vi "Teleop.vi"(10 "Match Info":T1={"Autonomous Elapsed Seconds"=0.0, "TeleOp Elapsed Seconds"=0.0, "Disabled Elapsed Seconds"=0.0, "Visited Autonomous"=FALSE, "Visited TeleOp"=FALSE, "Visited Disabled"=FALSE, "Autonomous Settings"={"Autonomous Style"=enum."Independent", "VI Refnum"=refnum}}, 11 "Call Context":T2) -> ()   [LabVIEW 2020]
doc: "This VI is called for each enabled TeleOp packet received from the DS. It is typically used to read from joysticks and other inputs and update I/O or setpoints for timed control loops. It should complete and return within 20 milliseconds or risk missing DS packets."
uses:
  <vilib>/Rock Robotics/WPI/DriverStation/WPI_DriverStationDerivedRobotMode.ctl
  <vilib>/Rock Robotics/WPI/DriverStation/WPI_DriverStationMatch Info.ctl
  <vilib>/Rock Robotics/WPI/ThirdParty/REV Robotics/REVLib/Typedef/Spark MAX Control Type.ctl
  <vilib>/Rock Robotics/WPI/Utilities/WPI_GetSetVariantRefNum.vi
  <vilib>/Rock Robotics/Network Tables/NT Write Boolean Array.vi
  <vilib>/Rock Robotics/Network Tables/NT Write Numeric Array.vi
  Framework/Robot Global Data.vi
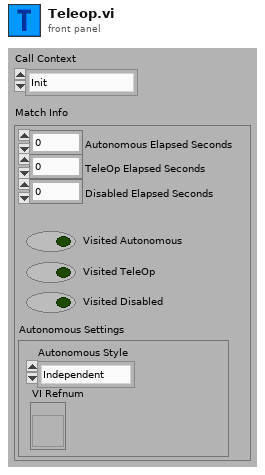
[diagram p1: front panel]
types:
  T1 = typedef "WPI_DriverStationMatch Info.ctl" = cluster{"Autonomous Elapsed Seconds":dbl, "TeleOp Elapsed Seconds":dbl, "Disabled Elapsed Seconds":dbl, "Visited Autonomous":bool, "Visited TeleOp":bool, "Visited Disabled":bool, "Autonomous Settings":cluster{"Autonomous Style":enum16{"Iterative", "Independent"}, "VI Refnum":refnum<vi>}}
  T2 = typedef "WPI_DriverStationDerivedRobotMode.ctl" = enum16{"Init", "Execute", "Stop"}
  T3 = typedef "Spark MAX Control Type.ctl" = enum16{"Percent VBus", "Voltage", "Velocity", "Position", "Smart Motion", "Current", "Smart Velocity"}
  T4 = typedef "WPI_JoystickDevRef.ctl" = cluster{"Device":T5}
  T5 = typedef "WPI_JoystickDeviceEnum.ctl" = enum16{"USB 0", "USB 1", "USB 2", "USB 3", "USB 4", "USB 5"}
  T6 = typedef "Command Status Info.ctl" = cluster{"Name":string, "Status":T7, "notifier out":T8}
  T7 = typedef "Completion Status.ctl" = enum16{"Successful", "Aborted", "Incomplete"}
  T8 = typedef "Completion Notifier.ctl" = refnum<notifier>
  T9 = typedef "WPI_MotorControlDeviceRef.ctl" = cluster{"DeviceStatus":errorcluster, "Type":T10, "PWM":cluster{"PWM Channel":T11, "DeadBand":T12}, "CAN":cluster{"Device Number":u8, "SetOutput VI Ref":variant, "GetOutput VI Ref":variant, "Enable VI Ref":variant, "Disable VI Ref":variant, "Data":variant}, "Invert":bool, "DIO PWM":cluster{"PWM \"Enable\" Channel":T11, "DIOChannel":T13, "PWM Rate":dbl}}
  T10 = typedef "WPI_MotorControlType.ctl" = enum16{"PWM", "CAN", "DIO PWM"}
  T11 = typedef "FPGA_DIOPWMChannel.ctl" = enum8{"PWM 0", "PWM 1", "PWM 2", "PWM 3", "PWM 4", "PWM 5", "PWM 6", "PWM 7", "PWM 8", "PWM 9", "PWM MXP 0", "PWM MXP 1", "PWM MXP 2", "PWM MXP 3", "PWM MXP 4", "PWM MXP 5", "PWM MXP 6", "PWM MXP 7", "PWM MXP 8", "PWM MXP 9", "Invalid"}
  T12 = typedef "WPI_PWMDeadband.ctl" = cluster{"Name":string, "maxPositivePwm":i32, "minPositivePwm":i32, "centerPwm":i32, "maxNegativePwm":i32, "minNegativePwm":i32, "angularRange":u16}
  T13 = typedef "FPGA_DIOChannel.ctl" = enum8{"DIO 0", "DIO 1", "DIO 2", "DIO 3", "DIO 4", "DIO 5", "DIO 6", "DIO 7", "DIO 8", "DIO 9", "DIO MXP 0", "DIO MXP 1", "DIO MXP 2", "DIO MXP 3", "DIO MXP 4", "DIO MXP 5", "DIO MXP 6", "DIO MXP 7", "DIO MXP 8", "DIO MXP 9", "DIO MXP 10", "DIO MXP 11", "DIO MXP 12", "DIO MXP 13", "DIO MXP 14", "DIO MXP 15", "SPI Port CS1", "SPI Port CS2", "SPI Port CS3", "SPI Port MISO", "SPI Port MOSI", "Invalid"}
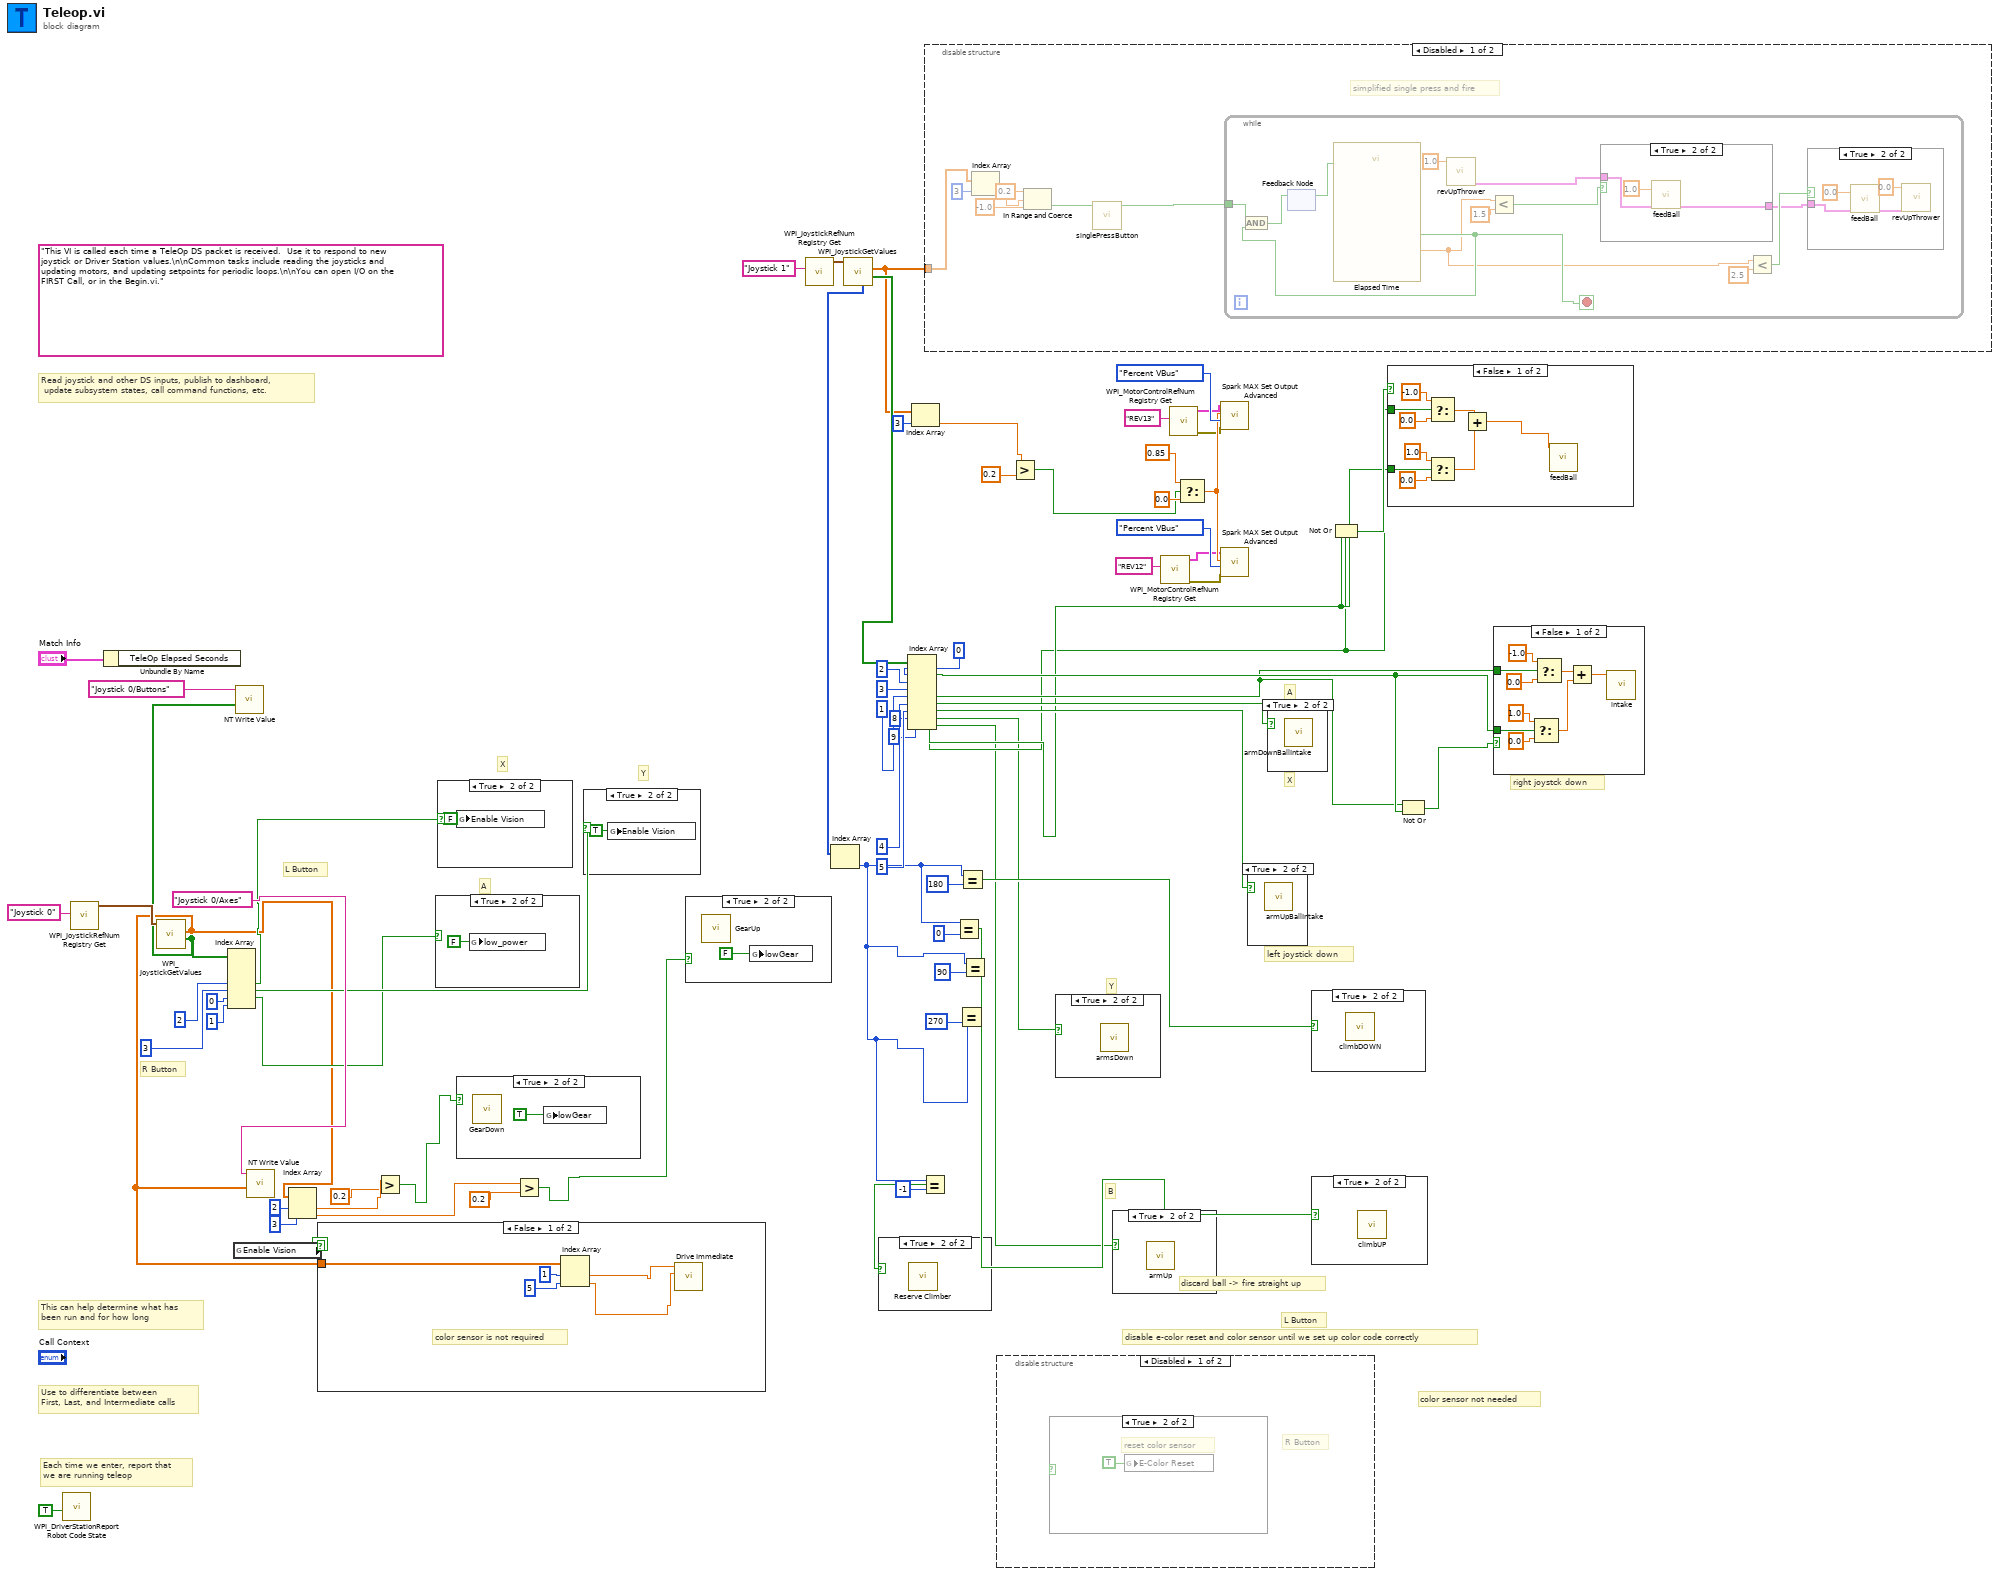
[diagram p0: block diagram]
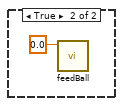
[diagram p9: hidden frame]
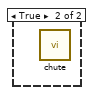
[diagram p18: hidden frame]
diagram:
  (unwired) "This VI is called each time a TeleOp DS packet is received.  Use it to respond to new joystick or Driver Station values.\n\nCommon tasks include reading the joysticks and updating motors, and updating setpoints for periodic loops.\n\nYou can open I/O on the FIRST Call, or in the Begin.vi."
  # "color sensor not needed"
  # "A"
  # "Y"
  # "X"
  # "disable e-color reset and color sensor until we set up color code correctly"
  # "right joystck down"
  # "left joystick down"
  # "B"
  # "Y"
  # "X"
  # "A"
  # "discard ball -> fire straight up"
  # "R Button"
  # "L Button"
  # "L Button"
  # "Read joystick and other DS inputs, publish to dashboard,\n update subsystem states, call command functions, etc."
  # "Each time we enter, report that\nwe are running teleop"
  # "Use to differentiate between\nFirst, Last, and Intermediate calls"
  # "This can help determine what has\nbeen run and for how long"
  n1 = call <vilib>:"WPI_DriverStationReport Robot Code State.vi"("TeleOp"=TRUE ("Autonomous")) -> ()  [unwired: 10 in, 1 out]
  n2 = call <vilib>:"WPI_JoystickRefNum Registry Get.vi"("refnum name"="Joystick 0") -> ("JoystickDevRef"=w68:T4)  [unwired: 1 in, 9 out]
  n3 = Unbundle By Name("Match Info") -> ()  [unwired: 1 out]
  n4 = call <vilib>:"WPI_JoystickGetValues.vi"("JoystickDevRef"=w68) -> ("Buttons"=w65:bool[], "Axes"=w24:dbl[])  [unwired: 6 in, 3 out]
  n5 = Index Array(array=w65, index #3=2 ("index"), index #4=3 ("index"), index #5=0 ("index"), index #6=1 ("index")) -> (element #3=w55:bool, element #4=w56:bool, element #5=w33:bool)  [unwired: 2 in, 3 out]
  n6 = global read "Robot Global Data.vi" "Enable Vision"() -> (w61:bool)
  n7 = call-poly <vilib>:"NT Write Value.vi"("Boolean Array"=w65, "Name"="Joystick 0/Buttons") -> ()  [unwired: 9 in, 1 out]
  n8 = call-poly <vilib>:"NT Write Value.vi"("Numeric Array"=w24, "Name"="Joystick 0/Axes") -> ()  [unwired: 9 in, 1 out]
  n9 = Index Array(array=w24, index #1=2 ("index"), index #2=3 ("index")) -> (element #1=w21:dbl, element #2=w17:dbl)
  n10 = case shown="False" w61 {
    tunnel: w24 -> [w76 _]
    frame False {
      # "color sensor is not required"
      n11 = Index Array(array=w76, index #1=1 ("index"), index #2=5 ("index")) -> (element #1=w73:dbl, element #2=w72:dbl)
      n12 = call "Drive Immediate.vi"("Right Setpoint"=w72, "Left Setpoint"=w73) -> ()  [unwired: 9 in, 1 out]
    }
    frame True {
    }
  }
  n13 = Greater?(x=w21, y=0.2 ("upper limit")) -> (0:w19:bool)
  n14 = case shown="True" w33 {
    frame False {
    }
    frame True {
      n15 = global write "Robot Global Data.vi" "low_power"(FALSE ("low_power")) -> ()
    }
  }
  n16 = case shown="True" w55 {
    frame False {
    }
    frame True {
      n17 = global write "Robot Global Data.vi" "Enable Vision"(FALSE ("Enable Vision")) -> ()
    }
  }
  n18 = case shown="True" w19 {
    frame False {
    }
    frame True {
      n19 = call "GearDown.vi"() -> ()  [unwired: 11 in, 1 out]
      n20 = global write "Robot Global Data.vi" "lowGear"(TRUE ("Enable Vision")) -> ()
    }
  }
  n21 = Greater?(x=w17, y=0.2 ("upper limit")) -> (0:w16:bool)
  n22 = case shown="True" w56 {
    frame False {
    }
    frame True {
      n23 = global write "Robot Global Data.vi" "Enable Vision"(TRUE ("Enable Vision")) -> ()
    }
  }
  n24 = case shown="True" w16 {
    frame False {
    }
    frame True {
      n25 = call "GearUp.vi"() -> ()  [unwired: 11 in, 1 out]
      n26 = global write "Robot Global Data.vi" "lowGear"(FALSE ("Enable Vision")) -> ()
    }
  }
  n27 = call <vilib>:"WPI_JoystickRefNum Registry Get.vi"("refnum name"="Joystick 1") -> ("JoystickDevRef"=w63:T4)  [unwired: 1 in, 9 out]
  n28 = call <vilib>:"WPI_JoystickGetValues.vi"("JoystickDevRef"=w63) -> ("Buttons"=w62:bool[], "Axes"=w4:dbl[], "POVs"=w50:i16[])  [unwired: 6 in, 2 out]
  n29 = Index Array(array=w50) -> (element=w32:i16)  [unwired: 1 in]
  n30 = Index Array(array=w62, index #1=0 ("index"), index #2=2 ("index"), index #3=3 ("index"), index #4=1 ("index"), index #5=4 ("index"), index #6=5 ("index"), index #7=8 ("index"), index #8=9 ("index")) -> (element #1=w39:bool, element #2=w36:bool, element #3=w35:bool, element #4=w38:bool, element #5=w42:bool, element #6=w41:bool, element #7=w26:bool, element #8=w25:bool)
  n31 = Index Array(array=w4, index=3) -> (element=w1:dbl)
  n32 = Equal?(x=w32, y=i16 -1) -> (x = y?=w30:bool)
  n33 = case shown="True" w30 {
    frame False {
    }
    frame True {
      n34 = call "Reserve Climber.vi"() -> ()  [unwired: 11 in, 1 out]
    }
  }
  n35 = disable-structure shown="Disabled" {
    disable-tunnel: w4 -> [w85 _]
    frame Disabled {
      # "simplified single press and fire"
      n36 = Index Array(array=w85, index=3) -> (element=w88:dbl)
      n37 = In Range and Coerce(upper limit=0.2, x=w88, lower limit=-1.0) -> (In Range?=w83:bool)  [unwired: 1 out]
      n38 = call "singlePressButton.vi"("Boolean"=w83) -> ("Boolean 2"=w82:bool)  [unwired: 10 in]
      n39 = while {
        tunnel: w82 -> [w100]
        stop <- w99 stop-if-true
        n40 = feedback #1() -> (w97:bool)  [unwired: 1 in]
        n41 = call "Elapsed Time"("Reset"=w97) -> ("Elapsed Time (s)"=w92:dbl, "Time has Elapsed"=w99:bool)  [unwired: 11 in, 6 out]
        n42 = And(x=w100, y=w99) -> (x .and. y?=w98:bool)
        n43 = feedback-in #1(w98) -> ()
        n44 = call "revUpThrower.vi"("Setpoint"=1.0) -> ("Command Info Out"=w94:T6)  [unwired: 10 in]
        n45 = Less?(x=w92, y=1.5) -> (x < y?=w95:bool)
        n46 = case shown="True" w95 {
          tunnel: w94 -> [_ w106]
          tunnel: [_ w105] -> w90
          frame False {
          }
          frame True {
            n47 = call "feedBall.vi"("Command Info In"=w106, "Setpoint"=1.0) -> ("Command Info Out"=w105:T6)  [unwired: 9 in]
          }
        }
        n48 = Less?(x=w92, y=2.5) -> (x < y?=w91:bool)
        n49 = case shown="True" w91 {
          tunnel: w90 -> [_ w103]
          frame False {
          }
          frame True {
            n50 = call "feedBall.vi"("Command Info In"=w103, "Setpoint"=0.0) -> ("Command Info Out"=w101:T6)  [unwired: 9 in]
            n51 = call "revUpThrower.vi"("Command Info In"=w101, "Setpoint"=0.0) -> ()  [unwired: 9 in, 1 out]
          }
        }
      }
    }
    frame Enabled {
    }
  }
  n52 = Equal?(x=w32, y=i16 0) -> (x = y?=w47:bool)
  n53 = Equal?(x=w32, y=i16 270) -> ()  [unwired: 1 out]
  n54 = Equal?(x=w32, y=i16 180) -> (x = y?=w29:bool)
  n55 = Equal?(x=w32, y=i16 90) -> ()  [unwired: 1 out]
  n56 = disable-structure shown="Disabled" {
    frame Disabled {
      # "R Button"
      n57 = case shown="True" {
        selector: _ -> [_ _]
        frame False {
        }
        frame True {
          # "reset color sensor"
          n58 = global write "Robot Global Data.vi" "E-Color Reset"(TRUE ("E-Color Reset")) -> ()
        }
      }
    }
    frame Enabled {
    }
  }
  n59 = Greater?(x=w1, y=0.2) -> (0:w2:bool)
  n60 = case shown="True" w26 {
    frame False {
    }
    frame True {
      n61 = call "armsDown.vi"() -> ()  [unwired: 11 in, 1 out]
    }
  }
  n62 = case shown="True" w25 {
    frame False {
    }
    frame True {
      n63 = call "armUp.vi"() -> ()  [unwired: 11 in, 1 out]
    }
  }
  n64 = call <vilib>:"WPI_MotorControlRefNum Registry Get.vi"("refnum name"="REV12") -> ("error out"=w9:errorcluster, "MotorControlDevRef"=w10:T9)  [unwired: 9 in]
  n65 = call <vilib>:"WPI_MotorControlRefNum Registry Get.vi"("refnum name"="REV13") -> ("error out"=w5:errorcluster, "MotorControlDevRef"=w6:T9)  [unwired: 9 in]
  n66 = Select(t=0.85, s=w2, f=0.0) -> (s? t:f=w11:dbl)
  n67 = call <vilib>:"Spark MAX Set Output Advanced.vi"("error in (no error)"=w5, "Control Mode"=Spark_MAX_Control_Type."Percent VBus", "Setpoint"=w11, "MotorControlDevRef"=w6) -> ()  [unwired: 6 in, 2 out]
  n68 = call <vilib>:"Spark MAX Set Output Advanced.vi"("error in (no error)"=w9, "Control Mode"=Spark_MAX_Control_Type."Percent VBus", "Setpoint"=w11, "MotorControlDevRef"=w10) -> ()  [unwired: 6 in, 2 out]
  n69 = case shown="True" w41 {
    frame False {
    }
    frame True {
      n70 = call "armUpBallIntake.vi"() -> ()  [unwired: 11 in, 1 out]
    }
  }
  n71 = case shown="True" w42 {
    frame False {
    }
    frame True {
      n72 = call "armDownBallIntake.vi"() -> ()  [unwired: 11 in, 1 out]
    }
  }
  n73 = case shown="True" w29 {
    frame False {
    }
    frame True {
      n74 = call "climbDOWN.vi"() -> ()  [unwired: 11 in, 1 out]
    }
  }
  n75 = case shown="True" w47 {
    frame False {
    }
    frame True {
      n76 = call "climbUP.vi"() -> ()  [unwired: 11 in, 1 out]
    }
  }
  n77 = Not Or(1:w36, 2:w35) -> (0:w37:bool)
  n78 = case shown="False" w37 {
    tunnel: w35 -> [w114 _]
    tunnel: w36 -> [w110 _]
    frame False {
      n79 = Select(t=-1.0, s=w114, f=0.0) -> (s? t:f=w112:dbl)
      n80 = Select(t=1.0, s=w110, f=0.0) -> (s? t:f=w111:dbl)
      n81 = Add(x=w112, y=w111) -> (x+y=w109:dbl)
      n82 = call "feedBall.vi"("Setpoint"=w109) -> ()  [unwired: 10 in, 1 out]
    }
    frame True {
      n83 = call "feedBall.vi"("Setpoint"=0.0) -> ()  [unwired: 10 in, 1 out]
    }
  }
  n84 = Not Or(1:w39, 2:w38) -> (0:w34:bool)
  n85 = case shown="False" w34 {
    tunnel: w39 -> [w126 _]
    tunnel: w38 -> [w123 _]
    frame False {
      n86 = Select(t=1.0, s=w126, f=0.0) -> (s? t:f=w120:dbl)
      n87 = Select(t=-1.0, s=w123, f=0.0) -> (s? t:f=w121:dbl)
      n88 = Add(x=w121, y=w120) -> (x+y=w119:dbl)
      n89 = call "intake.vi"("Setpoint"=w119) -> ()  [unwired: 10 in, 1 out]
    }
    frame True {
      n90 = call "chute.vi"() -> ()  [unwired: 11 in, 1 out]
    }
  }
